vi "Replace Scheme Color.vi"(6 "Theme Mode":u16(ring) items=["Light Theme", "Light Medium Contrast", "Light High Contrast", "Dark Theme", "Dark Medium Contrast", "Dark High Constrast"], 8 "Colorbox ref in":refnum<vi>, 9 "This VI":refnum<vi>, 10 "TabControl in":refnum<vi>, 11 "Material Theme in":refnum<class "Material Theme.lvclass">) -> (3 "Material Theme out":refnum<class "Material Theme.lvclass">)   [LabVIEW 2021, in "TSC Material Theme.lvlib" / "Material Theme.lvclass"]
doc: "This VI will grab the information for which color box was clicked on in the material theme editor UI and apply it to the given scheme that has selected for the overall file. This allows for propagated updates when the theme is resaved and reloaded.\n\n<b>Code Developed By:</b> +\nDaniel Coons +\nhttps://github.com/danielcoons/"
uses:
  Material Theme.lvclass
  _Material Theme SubVIs/scheme--enum.ctl
  Material Theme.lvclass/Material Theme.ctl
  Material-Scheme/Material-Scheme.lvclass/Material-Scheme.ctl
  Material-Scheme/data member access/Set primary.vi
  Material-Scheme/data member access/Set surfaceTint.vi
  Material-Scheme/data member access/Set onPrimary.vi
  Material-Scheme/data member access/Set primaryContainer.vi
  Material-Scheme/data member access/Set onPrimaryContainer.vi
  Material-Scheme/data member access/Set secondary.vi
  Material-Scheme/data member access/Set onSecondary.vi
  Material-Scheme/data member access/Set secondaryContainer.vi
  Material-Scheme/data member access/Set onSecondaryContainer.vi
  Material-Scheme/data member access/Set tertiary.vi
  Material-Scheme/data member access/Set onTertiary.vi
  Material-Scheme/data member access/Set tertiaryContainer.vi
  Material-Scheme/data member access/Set onTertiaryContainer.vi
  Material-Scheme/data member access/Set error.vi
  Material-Scheme/data member access/Set onError.vi
  Material-Scheme/data member access/Set errorContainer.vi
  Material-Scheme/data member access/Set onErrorContainer.vi
  Material-Scheme/data member access/Set background.vi
  Material-Scheme/data member access/Set onBackground.vi
  Material-Scheme/data member access/Set surface.vi
  Material-Scheme/data member access/Set onSurface.vi
  Material-Scheme/data member access/Set surfaceVariant.vi
  Material-Scheme/data member access/Set onSurfaceVariant.vi
  Material-Scheme/data member access/Set outline.vi
  Material-Scheme/data member access/Set outlineVariant.vi
  Material-Scheme/data member access/Set shadow.vi
  Material-Scheme/data member access/Set scrim.vi
  Material-Scheme/data member access/Set inverseSurface.vi
  Material-Scheme/data member access/Set inverseOnSurface.vi
  Material-Scheme/data member access/Set inversePrimary.vi
  Material-Scheme/data member access/Set primaryFixed.vi
  Material-Scheme/data member access/Set onPrimaryFixed.vi
  Material-Scheme/data member access/Set primaryFixedDim.vi
  Material-Scheme/data member access/Set onPrimaryFixedVariant.vi
  Material-Scheme/data member access/Set secondaryFixed.vi
  Material-Scheme/data member access/Set onSecondaryFixed.vi
  Material-Scheme/data member access/Set secondaryFixedDim.vi
  Material-Scheme/data member access/Set onSecondaryFixedVariant.vi
  Material-Scheme/data member access/Set tertiaryFixed.vi
  Material-Scheme/data member access/Set onTertiaryFixed.vi
  Material-Scheme/data member access/Set tertiaryFixedDim.vi
  Material-Scheme/data member access/Set onTertiaryFixedVariant.vi
  Material-Scheme/data member access/Set surfaceDim.vi
  Material-Scheme/data member access/Set surfaceBright.vi
  Material-Scheme/data member access/Set surfaceContainerLowest.vi
  Material-Scheme/data member access/Set surfaceContainerLow.vi
  Material-Scheme/data member access/Set surfaceContainer.vi
  Material-Scheme/data member access/Set surfaceContainerHigh.vi
  Material-Scheme/data member access/Set surfaceContainerHighest.vi
  Material-Scheme/Material-Scheme.lvclass
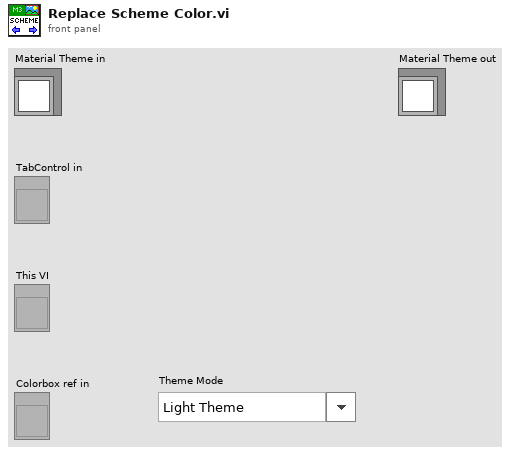
[diagram p1: front panel]
types:
  T1 = typedef "scheme--enum.ctl" = enum16{"primary", "surfacetint", "onprimary", "primarycontainer", "onprimarycontainer", "secondary", "onsecondary", "secondarycontainer", "onsecondarycontainer", "tertiary", "ontertiary", "tertiarycontainer", "ontertiarycontainer", "error", "onerror", "errorcontainer", "onerrorcontainer", "background", "onbackground", "surface", "onsurface", "surfacevariant", "onsurfacevar", "outline", "outlinevariant", "shadow", "scrim", "inversesurface", "inverseonsurface", "inverseprimary", "primaryfixed", "onprimaryfixed", "primaryfixeddim", "onprimaryfixedvariant", "secondaryfixed", "onsecondaryfixed", "secondaryfixeddim", "onsecondaryfixedvariant", "tertiaryfixed", "ontertiaryfixed", "tertiaryfixeddim", "ontertiartyfixedvariant", "surfacedim", "surfacebright", "surfcontainerlowest", "surfcontainerlow", "surfcontainer", "surfcontainerhigh", "surfcontainerhighest"}
  T2 = typedef "LVRectTypeDef.ctl" = cluster{"Left":i16, "Top":i16, "Right":i16, "Bottom":i16}
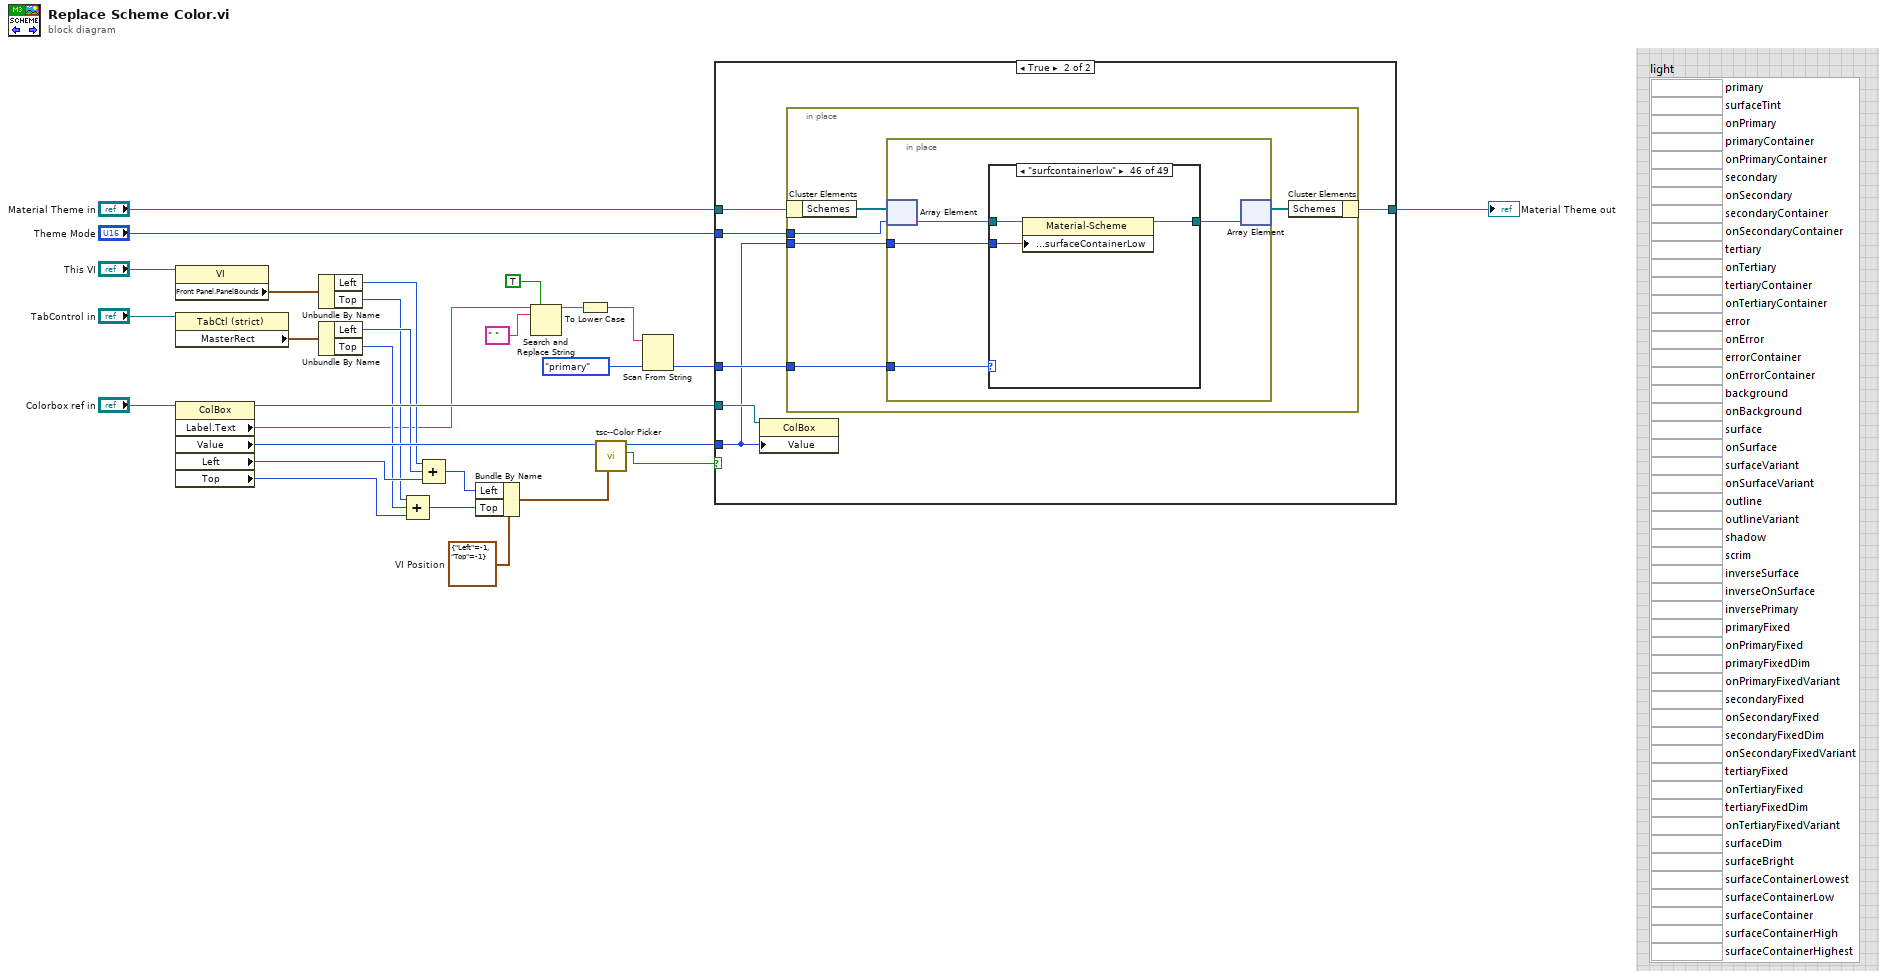
[diagram p0: block diagram]
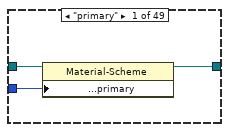
[diagram p3: hidden frame]
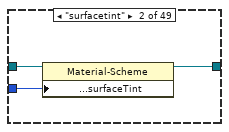
[diagram p4: hidden frame]
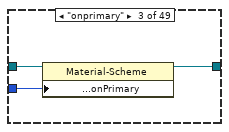
[diagram p5: hidden frame]
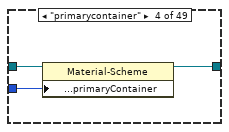
[diagram p6: hidden frame]
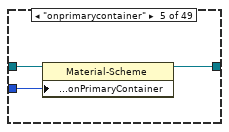
[diagram p7: hidden frame]
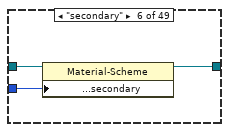
[diagram p8: hidden frame]
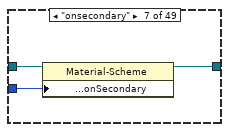
[diagram p9: hidden frame]
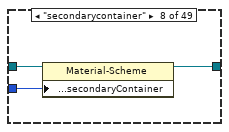
[diagram p10: hidden frame]
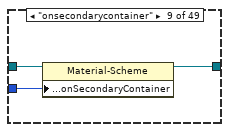
[diagram p11: hidden frame]
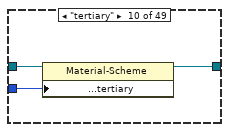
[diagram p12: hidden frame]
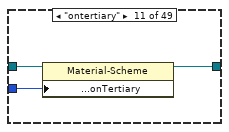
[diagram p13: hidden frame]
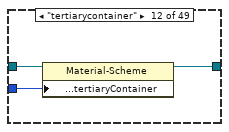
[diagram p14: hidden frame]
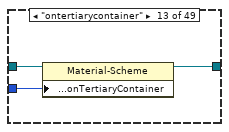
[diagram p15: hidden frame]
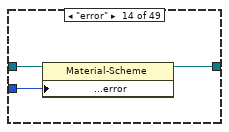
[diagram p16: hidden frame]
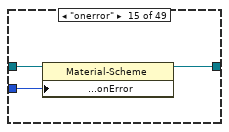
[diagram p17: hidden frame]
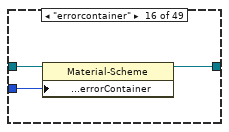
[diagram p18: hidden frame]
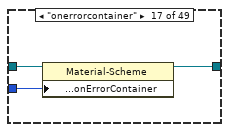
[diagram p19: hidden frame]
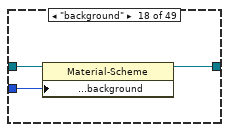
[diagram p20: hidden frame]
diagram:
  w22 = cluster{"Left":i16, "Top":i16} {"Left"=-1, "Top"=-1}  # VI Position
  n1 = property class="VI"(reference="This VI") -> ("Front Panel.PanelBounds"=w14:T2)  [unwired: 1 in, 2 out]
  n2 = property on="Property Node" class="TabCtl (strict)"(reference="TabControl in") -> ("MasterRect"=w17:T2)  [unwired: 1 in, 2 out]
  n3 = property class="ColBox"(reference="Colorbox ref in") -> (reference out=w26:refnum<vi>, "Label.Text"=w5:string, "Value"=w25:u32, "Left"=w19:i32, "Top"=w18:i32)  [unwired: 1 in, 1 out]
  n4 = Unbundle By Name(w14) -> ("Left"=w13:i16, "Top"=w12:i16)
  n5 = Unbundle By Name(w17) -> ("Left"=w16:i16, "Top"=w15:i16)
  n6 = Compound Arithmetic op=ADD(w12, w15, w18) -> (w11:i32)
  n7 = Compound Arithmetic op=ADD(w13, w16, w19) -> (w20:i32)
  n8 = Bundle By Name(cluster=w22, "Left"=w20, "Top"=w11) -> (w21:cluster{"Left":i16, "Top":i16})
  n9 = Search and Replace String(replace all?=TRUE ("replace all? (F)"), input string=w5, search string=" ") -> (result string=w4:string)  [unwired: 5 in, 3 out]
  n10 = To Lower Case(string=w4) -> (all lower case string=w1:string)
  n11 = call "tsc--Color Picker.vi"("VI Position"=w21, "input"=w25) -> ("accepted?"=w23:bool, "Resolved Color"=w24:u32)  [unwired: 8 in]
  n12 = Scan From String(input string=w1, default 1=scheme--enum."primary" ("scheme colors")) -> (output 1=w6:T1)  [unwired: 3 in, 3 out]
  n13 = case shown="True" w23 {
    tunnel: w24 -> [_ w31]
    tunnel: w26 -> [_ w36]
    tunnel: [w30 w34] -> w10
    tunnel: "Material Theme in" -> [w30 w35]
    tunnel: "Theme Mode" -> [_ w33]
    tunnel: w6 -> [_ w32]
    frame False {
    }
    frame True {
      n14 = property class="ColBox"(reference=w36, "Value"=w31) -> ()  [unwired: 1 in, 2 out]
      n15 = in-place {
        in-place-border: w33 -> [w40]
        in-place-border: w32 -> [w38]
        in-place-border: w31 -> [w37]
        n16 = in-place-cluster #1(w35) -> ("Schemes"=w41:refnum<class "Material-Scheme.lvclass">[])
        n17 = in-place {
          in-place-border: w38 -> [w43]
          in-place-border: w37 -> [w42]
          n18 = in-place-array #2(w41, w40) -> (w45:refnum<class "Material-Scheme.lvclass">)
          n19 = case shown="\"surfcontainerlow\"" w43 {
            tunnel: w45 -> [w48 w51 w54 w57 w60 w63 w66 w69 w72 w75 w78 w81 w84 w87 w90 w93 w96 w99 w102 w105 w108 w111 w114 w117 w120 w123 w126 w129 w132 w135 w138 w141 w144 w147 w150 w153 w156 w159 w162 w165 w168 w171 w174 w177 w180 w183 w186 w189 w192]
            tunnel: [w47 w50 w53 w56 w59 w62 w65 w68 w71 w74 w77 w80 w83 w86 w89 w92 w95 w98 w101 w104 w107 w110 w113 w116 w119 w122 w125 w128 w131 w134 w137 w140 w143 w146 w149 w152 w155 w158 w161 w164 w167 w170 w173 w176 w179 w182 w185 w188 w191] -> w44
            tunnel: w42 -> [w46 w49 w52 w55 w58 w61 w64 w67 w70 w73 w76 w79 w82 w85 w88 w91 w94 w97 w100 w103 w106 w109 w112 w115 w118 w121 w124 w127 w130 w133 w136 w139 w142 w145 w148 w151 w154 w157 w160 w163 w166 w169 w172 w175 w178 w181 w184 w187 w190]
            frame "primary" {
              n20 = property class="Material-Scheme"(reference=w48, "data member access:Theme Colors:primary"=w46) -> (reference out=w47:refnum<class "Material-Scheme.lvclass">)  [unwired: 1 in, 1 out]
            }
            frame "surfacetint" {
              n21 = property class="Material-Scheme"(reference=w51, "data member access:Surface:surfaceTint"=w49) -> (reference out=w50:refnum<class "Material-Scheme.lvclass">)  [unwired: 1 in, 1 out]
            }
            frame "onprimary" {
              n22 = property class="Material-Scheme"(reference=w54, "data member access:Text Colors:onPrimary"=w52) -> (reference out=w53:refnum<class "Material-Scheme.lvclass">)  [unwired: 1 in, 1 out]
            }
            frame "primarycontainer" {
              n23 = property class="Material-Scheme"(reference=w57, "data member access:Theme Colors:primaryContainer"=w55) -> (reference out=w56:refnum<class "Material-Scheme.lvclass">)  [unwired: 1 in, 1 out]
            }
            frame "onprimarycontainer" {
              n24 = property class="Material-Scheme"(reference=w60, "data member access:Text Colors:onPrimaryContainer"=w58) -> (reference out=w59:refnum<class "Material-Scheme.lvclass">)  [unwired: 1 in, 1 out]
            }
            frame "secondary" {
              n25 = property class="Material-Scheme"(reference=w63, "data member access:Theme Colors:secondary"=w61) -> (reference out=w62:refnum<class "Material-Scheme.lvclass">)  [unwired: 1 in, 1 out]
            }
            frame "onsecondary" {
              n26 = property class="Material-Scheme"(reference=w66, "data member access:Text Colors:onSecondary"=w64) -> (reference out=w65:refnum<class "Material-Scheme.lvclass">)  [unwired: 1 in, 1 out]
            }
            frame "secondarycontainer" {
              n27 = property class="Material-Scheme"(reference=w69, "data member access:Theme Colors:secondaryContainer"=w67) -> (reference out=w68:refnum<class "Material-Scheme.lvclass">)  [unwired: 1 in, 1 out]
            }
            frame "onsecondarycontainer" {
              n28 = property class="Material-Scheme"(reference=w72, "data member access:Text Colors:onSecondaryContainer"=w70) -> (reference out=w71:refnum<class "Material-Scheme.lvclass">)  [unwired: 1 in, 1 out]
            }
            frame "tertiary" {
              n29 = property class="Material-Scheme"(reference=w75, "data member access:Theme Colors:tertiary"=w73) -> (reference out=w74:refnum<class "Material-Scheme.lvclass">)  [unwired: 1 in, 1 out]
            }
            frame "ontertiary" {
              n30 = property class="Material-Scheme"(reference=w78, "data member access:Text Colors:onTertiary"=w76) -> (reference out=w77:refnum<class "Material-Scheme.lvclass">)  [unwired: 1 in, 1 out]
            }
            frame "tertiarycontainer" {
              n31 = property class="Material-Scheme"(reference=w81, "data member access:Theme Colors:tertiaryContainer"=w79) -> (reference out=w80:refnum<class "Material-Scheme.lvclass">)  [unwired: 1 in, 1 out]
            }
            frame "ontertiarycontainer" {
              n32 = property class="Material-Scheme"(reference=w84, "data member access:Text Colors:onTertiaryContainer"=w82) -> (reference out=w83:refnum<class "Material-Scheme.lvclass">)  [unwired: 1 in, 1 out]
            }
            frame "error" {
              n33 = property class="Material-Scheme"(reference=w87, "data member access:Theme Colors:error"=w85) -> (reference out=w86:refnum<class "Material-Scheme.lvclass">)  [unwired: 1 in, 1 out]
            }
            frame "onerror" {
              n34 = property class="Material-Scheme"(reference=w90, "data member access:Text Colors:onError"=w88) -> (reference out=w89:refnum<class "Material-Scheme.lvclass">)  [unwired: 1 in, 1 out]
            }
            frame "errorcontainer" {
              n35 = property class="Material-Scheme"(reference=w93, "data member access:Theme Colors:errorContainer"=w91) -> (reference out=w92:refnum<class "Material-Scheme.lvclass">)  [unwired: 1 in, 1 out]
            }
            frame "onerrorcontainer" {
              n36 = property class="Material-Scheme"(reference=w96, "data member access:Text Colors:onErrorContainer"=w94) -> (reference out=w95:refnum<class "Material-Scheme.lvclass">)  [unwired: 1 in, 1 out]
            }
            frame "background" {
              n37 = property class="Material-Scheme"(reference=w99, "data member access:Surface:background"=w97) -> (reference out=w98:refnum<class "Material-Scheme.lvclass">)  [unwired: 1 in, 1 out]
            }
            frame "onbackground" {
              n38 = property class="Material-Scheme"(reference=w102, "data member access:Text Colors:onBackground"=w100) -> (reference out=w101:refnum<class "Material-Scheme.lvclass">)  [unwired: 1 in, 1 out]
            }
            frame "surface" {
              n39 = property class="Material-Scheme"(reference=w105, "data member access:Surface:surface"=w103) -> (reference out=w104:refnum<class "Material-Scheme.lvclass">)  [unwired: 1 in, 1 out]
            }
            frame "onsurface" {
              n40 = property class="Material-Scheme"(reference=w108, "data member access:Text Colors:onSurface"=w106) -> (reference out=w107:refnum<class "Material-Scheme.lvclass">)  [unwired: 1 in, 1 out]
            }
            frame "surfacevariant" {
              n41 = property class="Material-Scheme"(reference=w111, "data member access:Surface:surfaceVariant"=w109) -> (reference out=w110:refnum<class "Material-Scheme.lvclass">)  [unwired: 1 in, 1 out]
            }
            frame "onsurfacevar" {
              n42 = property class="Material-Scheme"(reference=w114, "data member access:Text Colors:onSurfaceVariant"=w112) -> (reference out=w113:refnum<class "Material-Scheme.lvclass">)  [unwired: 1 in, 1 out]
            }
            frame "outline" {
              n43 = property class="Material-Scheme"(reference=w117, "data member access:Other:outline"=w115) -> (reference out=w116:refnum<class "Material-Scheme.lvclass">)  [unwired: 1 in, 1 out]
            }
            frame "outlinevariant" {
              n44 = property class="Material-Scheme"(reference=w120, "data member access:Other:outlineVariant"=w118) -> (reference out=w119:refnum<class "Material-Scheme.lvclass">)  [unwired: 1 in, 1 out]
            }
            frame "shadow" {
              n45 = property class="Material-Scheme"(reference=w123, "data member access:Other:shadow"=w121) -> (reference out=w122:refnum<class "Material-Scheme.lvclass">)  [unwired: 1 in, 1 out]
            }
            frame "scrim" {
              n46 = property class="Material-Scheme"(reference=w126, "data member access:Other:scrim"=w124) -> (reference out=w125:refnum<class "Material-Scheme.lvclass">)  [unwired: 1 in, 1 out]
            }
            frame "inversesurface" {
              n47 = property class="Material-Scheme"(reference=w129, "data member access:Surface:inverseSurface"=w127) -> (reference out=w128:refnum<class "Material-Scheme.lvclass">)  [unwired: 1 in, 1 out]
            }
            frame "inverseonsurface" {
              n48 = property class="Material-Scheme"(reference=w132, "data member access:Text Colors:inverseOnSurface"=w130) -> (reference out=w131:refnum<class "Material-Scheme.lvclass">)  [unwired: 1 in, 1 out]
            }
            frame "inverseprimary" {
              n49 = property class="Material-Scheme"(reference=w135, "data member access:Theme Colors:inversePrimary"=w133) -> (reference out=w134:refnum<class "Material-Scheme.lvclass">)  [unwired: 1 in, 1 out]
            }
            frame "primaryfixed" {
              n50 = property class="Material-Scheme"(reference=w138, "data member access:Fixed Colors:primaryFixed"=w136) -> (reference out=w137:refnum<class "Material-Scheme.lvclass">)  [unwired: 1 in, 1 out]
            }
            frame "onprimaryfixed" {
              n51 = property class="Material-Scheme"(reference=w141, "data member access:Text Colors Fixed:onPrimaryFixed"=w139) -> (reference out=w140:refnum<class "Material-Scheme.lvclass">)  [unwired: 1 in, 1 out]
            }
            frame "primaryfixeddim" {
              n52 = property class="Material-Scheme"(reference=w144, "data member access:Fixed Colors:primaryFixedDim"=w142) -> (reference out=w143:refnum<class "Material-Scheme.lvclass">)  [unwired: 1 in, 1 out]
            }
            frame "onprimaryfixedvariant" {
              n53 = property class="Material-Scheme"(reference=w147, "data member access:Text Colors Fixed:onPrimaryFixedVariant"=w145) -> (reference out=w146:refnum<class "Material-Scheme.lvclass">)  [unwired: 1 in, 1 out]
            }
            frame "secondaryfixed" {
              n54 = property class="Material-Scheme"(reference=w150, "data member access:Fixed Colors:secondaryFixed"=w148) -> (reference out=w149:refnum<class "Material-Scheme.lvclass">)  [unwired: 1 in, 1 out]
            }
            frame "onsecondaryfixed" {
              n55 = property class="Material-Scheme"(reference=w153, "data member access:Text Colors Fixed:onSecondaryFixed"=w151) -> (reference out=w152:refnum<class "Material-Scheme.lvclass">)  [unwired: 1 in, 1 out]
            }
            frame "secondaryfixeddim" {
              n56 = property class="Material-Scheme"(reference=w156, "data member access:Fixed Colors:secondaryFixedDim"=w154) -> (reference out=w155:refnum<class "Material-Scheme.lvclass">)  [unwired: 1 in, 1 out]
            }
            frame "onsecondaryfixedvariant" {
              n57 = property class="Material-Scheme"(reference=w159, "data member access:Text Colors Fixed:onSecondaryFixedVariant"=w157) -> (reference out=w158:refnum<class "Material-Scheme.lvclass">)  [unwired: 1 in, 1 out]
            }
            frame "tertiaryfixed" {
              n58 = property class="Material-Scheme"(reference=w162, "data member access:Fixed Colors:tertiaryFixed"=w160) -> (reference out=w161:refnum<class "Material-Scheme.lvclass">)  [unwired: 1 in, 1 out]
            }
            frame "ontertiaryfixed" {
              n59 = property class="Material-Scheme"(reference=w165, "data member access:Text Colors Fixed:onTertiaryFixed"=w163) -> (reference out=w164:refnum<class "Material-Scheme.lvclass">)  [unwired: 1 in, 1 out]
            }
            frame "tertiaryfixeddim" {
              n60 = property class="Material-Scheme"(reference=w168, "data member access:Fixed Colors:tertiaryFixedDim"=w166) -> (reference out=w167:refnum<class "Material-Scheme.lvclass">)  [unwired: 1 in, 1 out]
            }
            frame "ontertiartyfixedvariant" {
              n61 = property class="Material-Scheme"(reference=w171, "data member access:Text Colors Fixed:onTertiaryFixedVariant"=w169) -> (reference out=w170:refnum<class "Material-Scheme.lvclass">)  [unwired: 1 in, 1 out]
            }
            frame "surfacedim" {
              n62 = property class="Material-Scheme"(reference=w174, "data member access:Surface:surfaceDim"=w172) -> (reference out=w173:refnum<class "Material-Scheme.lvclass">)  [unwired: 1 in, 1 out]
            }
            frame "surfacebright" {
              n63 = property class="Material-Scheme"(reference=w177, "data member access:Surface:surfaceBright"=w175) -> (reference out=w176:refnum<class "Material-Scheme.lvclass">)  [unwired: 1 in, 1 out]
            }
            frame "surfcontainerlowest" {
              n64 = property class="Material-Scheme"(reference=w180, "data member access:Surface:surfaceContainerLowest"=w178) -> (reference out=w179:refnum<class "Material-Scheme.lvclass">)  [unwired: 1 in, 1 out]
            }
            frame "surfcontainerlow" {
              n65 = property class="Material-Scheme"(reference=w183, "data member access:Surface:surfaceContainerLow"=w181) -> (reference out=w182:refnum<class "Material-Scheme.lvclass">)  [unwired: 1 in, 1 out]
            }
            frame "surfcontainer" {
              n66 = property class="Material-Scheme"(reference=w186, "data member access:Surface:surfaceContainer"=w184) -> (reference out=w185:refnum<class "Material-Scheme.lvclass">)  [unwired: 1 in, 1 out]
            }
            frame "surfcontainerhigh" {
              n67 = property class="Material-Scheme"(reference=w189, "data member access:Surface:surfaceContainerHigh"=w187) -> (reference out=w188:refnum<class "Material-Scheme.lvclass">)  [unwired: 1 in, 1 out]
            }
            frame "surfcontainerhighest" {
              n68 = property class="Material-Scheme"(reference=w192, "data member access:Surface:surfaceContainerHighest"=w190) -> (reference out=w191:refnum<class "Material-Scheme.lvclass">)  [unwired: 1 in, 1 out]
            }
          }
          n69 = in-place-array #2(w44) -> (w39:refnum<class "Material-Scheme.lvclass">[])  [unwired: 1 out]
        }
        n70 = in-place-cluster #1("Schemes"=w39) -> (w34:refnum<class "Material Theme.lvclass">)
      }
    }
  }
  "Material Theme out" <- w10
